vi "Teleop.vi"(10 "Match Info":T2={"Autonomous Elapsed Seconds"=0.0, "TeleOp Elapsed Seconds"=0.0, "Disabled Elapsed Seconds"=0.0, "Visited Autonomous"=FALSE, "Visited TeleOp"=FALSE, "Visited Disabled"=FALSE, "Autonomous Settings"={"Autonomous Style"=enum."Independent", "VI Refnum"=refnum}}, 11 "Call Context":T3) -> ()   [LabVIEW 2015]
doc: "This VI is called for each TeleOp packet received from the DS where the robot is not disabled. It is often used to read from the joysticks and update I/O or to update setpoints for timed control loops. It should complete and return within 20 milliseconds or it may miss DS packets."
uses:
  <vilib>/Rock Robotics/WPI/DriverStation/WPI_DriverStationDerivedRobotMode.ctl
  <vilib>/Rock Robotics/WPI/DriverStation/WPI_DriverStationMatch Info.ctl
  <vilib>/Rock Robotics/WPI/CAN/TalonSRX/WPI_CANTalonSRX_GlobalStatus.ctl
  <vilib>/Rock Robotics/WPI/CAN/TalonSRX/WPI_CANTalonSRX_APIControlMode.ctl
  <vilib>/Rock Robotics/WPI/CAN/TalonSRX/WPI_CANTalonSRX_BrakeOverride.ctl
  <vilib>/Rock Robotics/WPI/Relay/WPI_RelayValue.ctl
  <vilib>/Rock Robotics/Network Tables/NT Write Boolean.vi
  <vilib>/Rock Robotics/WPI/Utilities/WPI_GetSetVariantRefNum.vi
  <vilib>/Rock Robotics/Network Tables/NT Read Boolean.vi
  <vilib>/Rock Robotics/WPI/Solenoid/WPI_SolenoidSetEnum.vi
  <vilib>/Rock Robotics/Network Tables/NT Write Numeric Array.vi
  <vilib>/Rock Robotics/Network Tables/NT Read Number.vi
  <vilib>/Rock Robotics/WPI/RobotDrive/WPI_RobotDriveArcadeDrive_Standard(NoSaturation).vi
panel:
  out "Encoder Position":dbl
  out "Left":T1
  out "Right":T1
  out "Talon SRX Status 2":T1
  out "Talon SRX Status":T1
  out "POSITION":dbl
  out "Theoretical Position":dbl
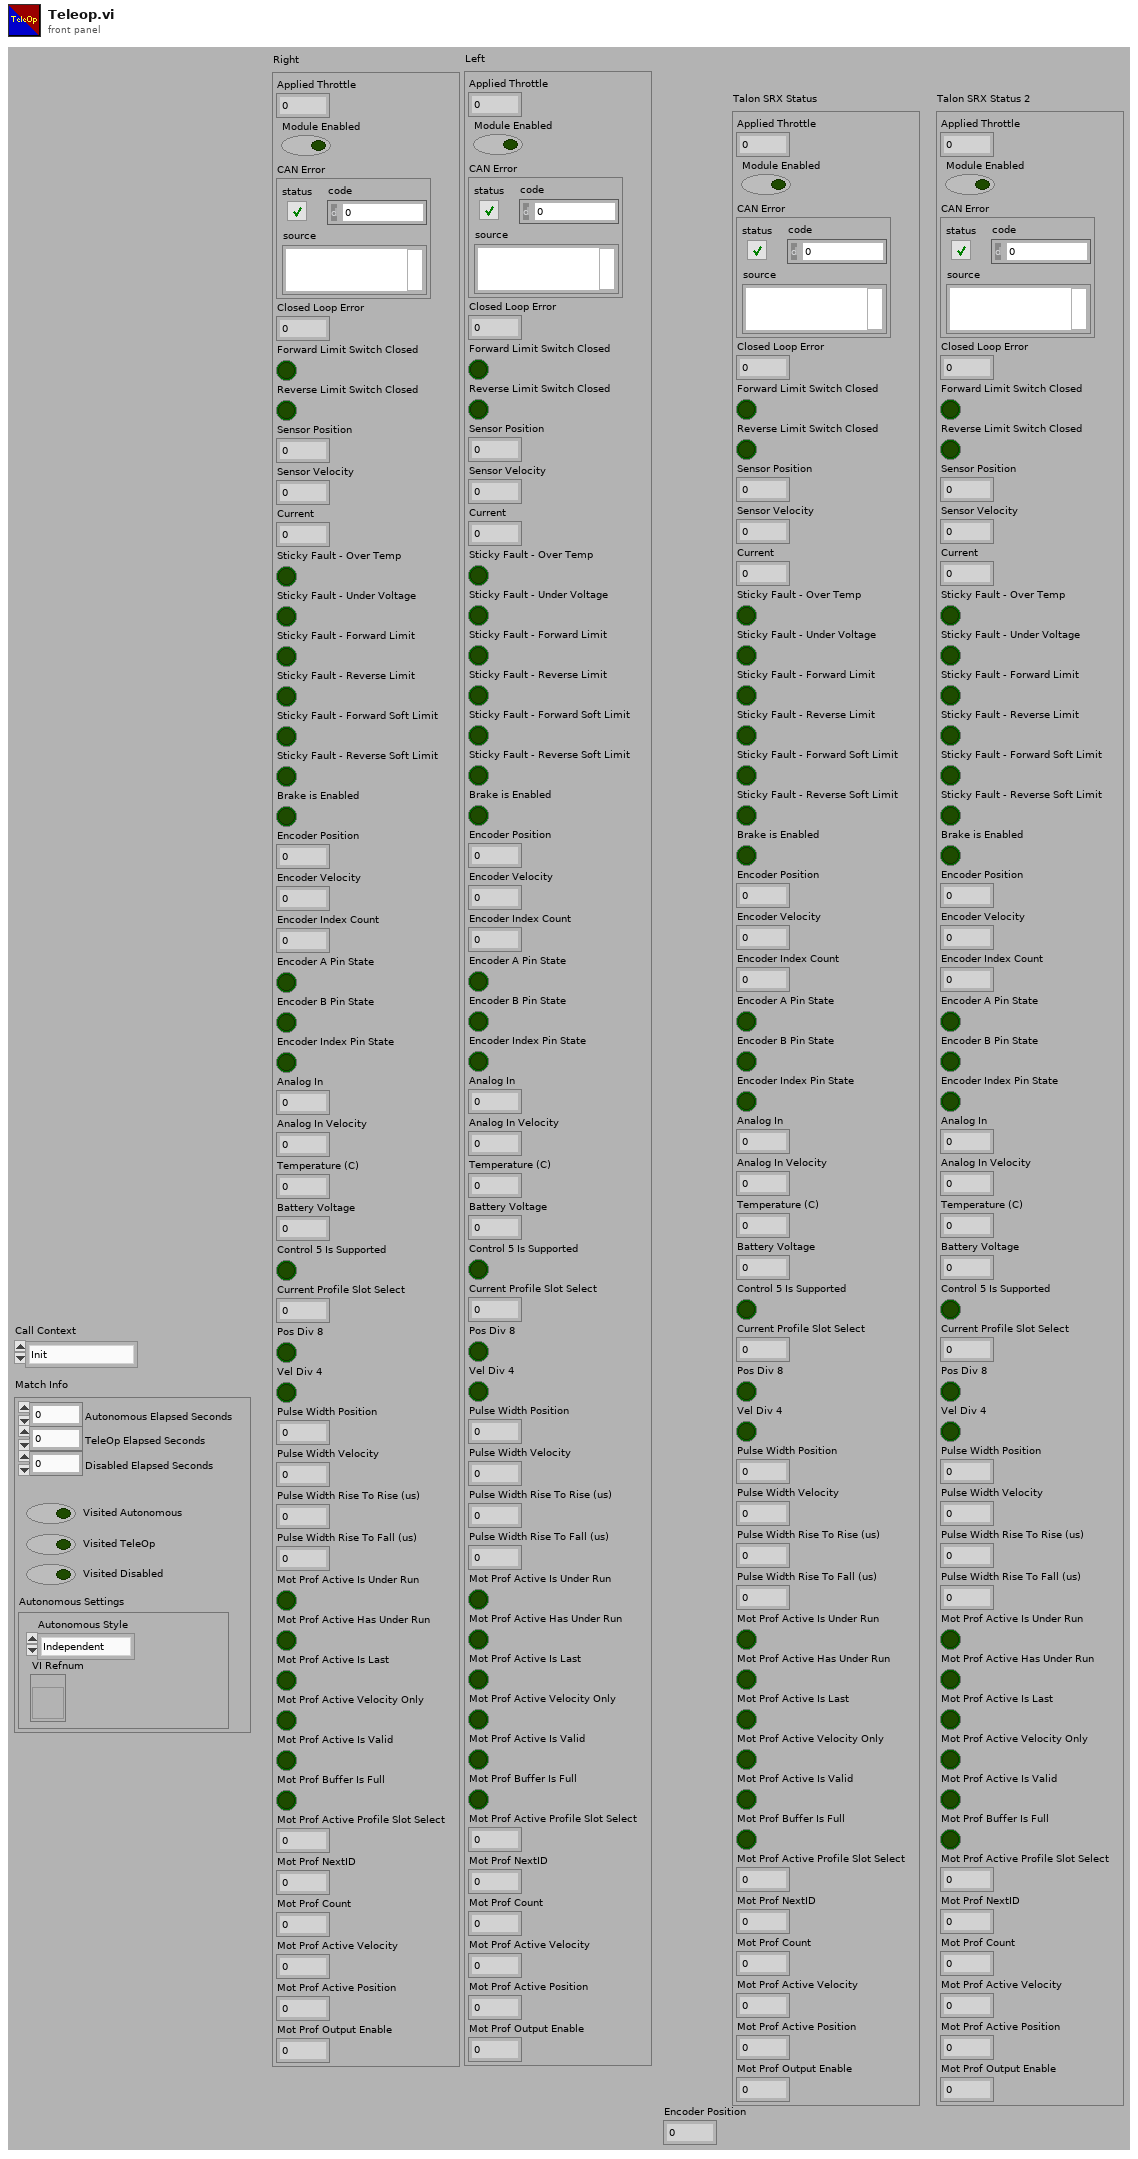
[diagram p1: front panel]
types:
  T1 = typedef "WPI_CANTalonSRX_GlobalStatus.ctl" = cluster{"Applied Throttle":dbl, "Module Enabled":bool, "CAN Error":errorcluster, "Closed Loop Error":dbl, "Forward Limit Switch Closed":bool, "Reverse Limit Switch Closed":bool, "Sensor Position":dbl, "Sensor Velocity":dbl, "Current":dbl, "Sticky Fault - Over Temp":bool, "Sticky Fault - Under Voltage":bool, "Sticky Fault - Forward Limit":bool, "Sticky Fault - Reverse Limit":bool, "Sticky Fault - Forward Soft Limit":bool, "Sticky Fault - Reverse Soft Limit":bool, "Brake is Enabled":bool, "Encoder Position":dbl, "Encoder Velocity":dbl, "Encoder Index Count":dbl, "Encoder A Pin State":bool, "Encoder B Pin State":bool, "Encoder Index Pin State":bool, "Analog In":dbl, "Analog In Velocity":dbl, "Temperature (C)":dbl, "Battery Voltage":dbl, "Control 5 Is Supported":bool, "Current Profile Slot Select":dbl, "Pos Div 8":bool, "Vel Div 4":bool, "Pulse Width Position":i32, "Pulse Width Velocity":i32, "Pulse Width Rise To Rise (us)":i32, "Pulse Width Rise To Fall (us)":i32, "Mot Prof Active Is Under Run":bool, "Mot Prof Active Has Under Run":bool, "Mot Prof Active Is Last":bool, "Mot Prof Active Velocity Only":bool, "Mot Prof Active Is Valid":bool, "Mot Prof Buffer Is Full":bool, "Mot Prof Active Profile Slot Select":i32, "Mot Prof NextID":i32, "Mot Prof Count":i32, "Mot Prof Active Velocity":dbl, "Mot Prof Active Position":dbl, "Mot Prof Output Enable":i32}
  T2 = typedef "WPI_DriverStationMatch Info.ctl" = cluster{"Autonomous Elapsed Seconds":dbl, "TeleOp Elapsed Seconds":dbl, "Disabled Elapsed Seconds":dbl, "Visited Autonomous":bool, "Visited TeleOp":bool, "Visited Disabled":bool, "Autonomous Settings":cluster{"Autonomous Style":enum16{"Iterative", "Independent"}, "VI Refnum":refnum<vi>}}
  T3 = typedef "WPI_DriverStationDerivedRobotMode.ctl" = enum16{"Init", "Execute", "Stop"}
  T4 = typedef "WPI_JoystickDevRef.ctl" = cluster{"Device":T5}
  T5 = typedef "WPI_JoystickDeviceEnum.ctl" = enum16{"USB 0", "USB 1", "USB 2", "USB 3", "USB 4", "USB 5"}
  T6 = cluster{"Axes[0]":dbl, "Axes[1]":dbl, "Axes[2]":dbl, "Axes[3]":dbl, "Axes[4]":dbl, "Axes[5]":dbl, "Axes[6]":dbl, "Axes[7]":dbl, "Axes[8]":dbl}
  T7 = cluster{"Buttons[0]":bool, "Buttons[1]":bool, "Buttons[2]":bool, "Buttons[3]":bool, "Buttons[4]":bool, "Buttons[5]":bool, "Buttons[6]":bool, "Buttons[7]":bool, "Buttons[8]":bool}
  T8 = typedef "WPI_RelayValue.ctl" = enum16{"Off", "On", "Forward", "Reverse"}
  T9 = typedef "WPI_ServoDeviceRef.ctl" = cluster{"DeviceStatus":errorcluster, "PWM Channel":T10, "DeadBand":T11}
  T10 = typedef "FPGA_DIOPWMChannel.ctl" = enum8{"PWM 0", "PWM 1", "PWM 2", "PWM 3", "PWM 4", "PWM 5", "PWM 6", "PWM 7", "PWM 8", "PWM 9", "PWM MXP 0", "PWM MXP 1", "PWM MXP 2", "PWM MXP 3", "PWM MXP 4", "PWM MXP 5", "PWM MXP 6", "PWM MXP 7", "PWM MXP 8", "PWM MXP 9", "Invalid"}
  T11 = typedef "WPI_PWMDeadband.ctl" = cluster{"Name":string, "maxPositivePwm":i32, "minPositivePwm":i32, "centerPwm":i32, "maxNegativePwm":i32, "minNegativePwm":i32, "angularRange":u16}
  T12 = typedef "WPI_SolenoidDevRef.ctl" = cluster{"DevStatus":errorcluster, "Pneumatics Control Module":u8, "Forward Solenoid Channel":T13, "Reverse Solenoid Channel":T13}
  T13 = typedef "WPI_SolenoidChannel.ctl" = enum8{"Solenoid 0", "Solenoid 1", "Solenoid 2", "Solenoid 3", "Solenoid 4", "Solenoid 5", "Solenoid 6", "Solenoid 7", "Invalid"}
  T14 = typedef "WPI_MotorControlDeviceRef.ctl" = cluster{"DeviceStatus":errorcluster, "Type":T15, "PWM":cluster{"PWM Channel":T10, "DeadBand":T11}, "CAN":cluster{"Device Number":u8, "Control Mode":T16, "Semaphore":T17, "Max Vout":dbl, "TalonSRX Control Mode":T18}, "Invert":bool}
  T15 = typedef "WPI_MotorControlType.ctl" = enum16{"PWM", "CAN", "CANTalonSRX"}
  T16 = typedef "WPI_CANJaguar_ControlMode.ctl" = enum8{"Percent VBus", "Current", "Speed", "Position", "Voltage"}
  T17 = typedef "Semaphore RefNum" = refnum<k1>
  T18 = typedef "WPI_CANTalonSRX_APIControlMode.ctl" = enum8{"Percent VBus", "Speed", "Position", "Slave", "Unchanged / Invalid", "Voltage Compensation", "Current", "Motion Profile"}
  T19 = typedef "WPI_CANTalonSRX_BrakeOverride.ctl" = enum8{"No Override", "Override to Coast", "Override to Brake"}
  T20 = typedef "WPI_RobotDriveDevRef.ctl" = cluster{"DevStatus":errorcluster, "Motors[]":T14[], "Square Inputs":bool, "Max Output":dbl}
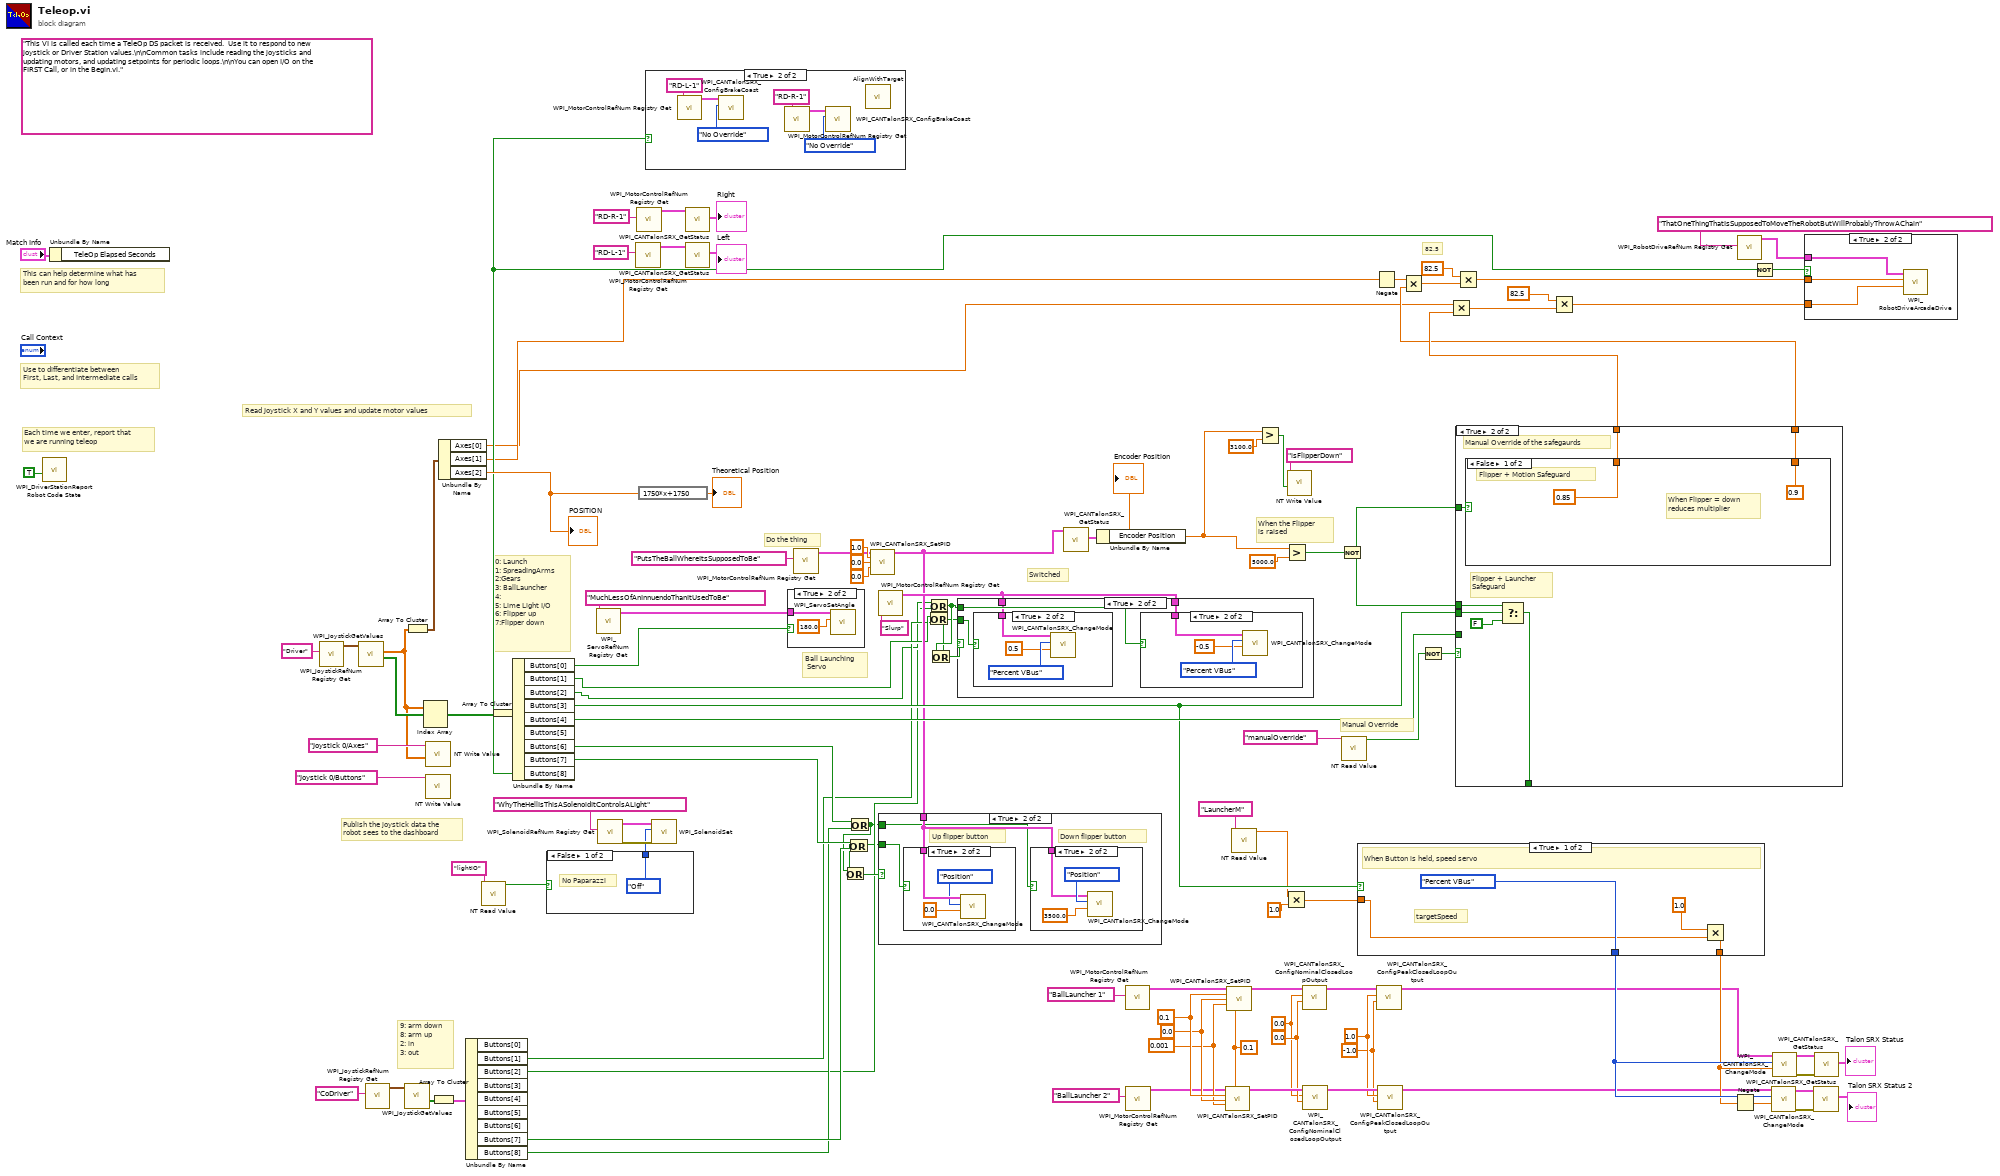
[diagram p0: block diagram]
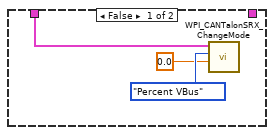
[diagram p7: hidden frame]
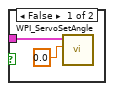
[diagram p10: hidden frame]
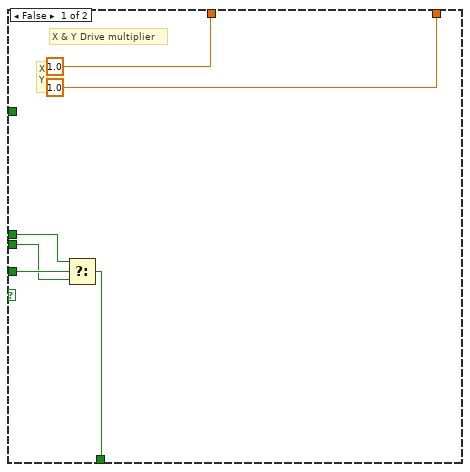
[diagram p11: hidden frame]
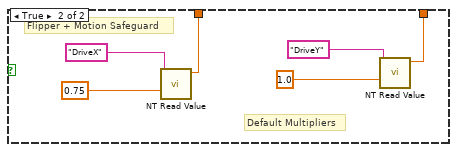
[diagram p12: hidden frame]
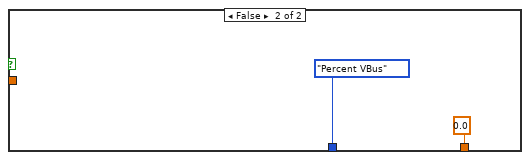
[diagram p13: hidden frame]
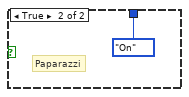
[diagram p14: hidden frame]
diagram:
  w33 = -1.0 ("Reverse Peak Output")
  w34 = 1.0 ("Forward Peak Output")
  w36 = 0.0 ("Reverse Nominal Output")
  w35 = 0.0 ("Forward Nominal Output")
  w32 = 0.1 ("F")
  w45 = 0.001 ("D")
  w46 = 0.0 ("I")
  w47 = 0.1 ("P")
  (unwired) "This VI is called each time a TeleOp DS packet is received.  Use it to respond to new joystick or Driver Station values.\n\nCommon tasks include reading the joysticks and updating motors, and updating setpoints for periodic loops.\n\nYou can open I/O on the FIRST Call, or in the Begin.vi."
  # "82.5"
  # "9: arm down\n8: arm up\n2: in \n3: out"
  # "Switched"
  # "Ball Launching\n Servo"
  # "Manual Override"
  # "When the Flipper \nis raised"
  # "0: Launch\n1: SpreadingArms\n2:Gears\n3: BallLauncher\n4: \n5: Lime Light I/O\n6: Flipper up\n7:Flipper down"
  # "Do the thing"
  # "Publish the joystick data the\nrobot sees to the dashboard"
  # "Read Joystick X and Y values and update motor values"
  # "Each time we enter, report that\nwe are running teleop"
  # "Use to differentiate between\nFirst, Last, and Intermediate calls"
  # "This can help determine what has\nbeen run and for how long"
  n1 = call <vilib>:"WPI_DriverStationReport Robot Code State.vi"("TeleOp"=TRUE ("Autonomous")) -> ()  [unwired: 10 in, 1 out]
  n2 = Unbundle By Name("Match Info") -> ()  [unwired: 1 out]
  n3 = call <vilib>:"WPI_JoystickRefNum Registry Get.vi"("refnum name"="Driver") -> ("JoystickDevRef"=w73:T4)  [unwired: 9 in, 1 out]
  n4 = call <vilib>:"WPI_JoystickGetValues.vi"("JoystickDevRef"=w73) -> ("Buttons"=w70:bool[], "Axes"=w69:dbl[])  [unwired: 6 in, 3 out]
  n5 = call <vilib>:"WPI_JoystickRefNum Registry Get.vi"("refnum name"="CoDriver") -> ("JoystickDevRef"=w21:T4)  [unwired: 9 in, 1 out]
  n6 = call <vilib>:"WPI_JoystickGetValues.vi"("JoystickDevRef"=w21) -> ("Buttons"=w19:bool[])  [unwired: 6 in, 4 out]
  n7 = Array To Cluster(array=w69) -> (cluster=w107:T6)
  n8 = Index Array(array=w69) -> ()  [unwired: 2 in, 2 out]
  n9 = call-poly <vilib>:"NT Write Value.vi"("Numeric Array"=w69, "Name"="Joystick 0/Axes") -> ()  [unwired: 9 in, 1 out]
  n10 = call-poly <vilib>:"NT Write Value.vi"("Name"="Joystick 0/Buttons") -> ()  [unwired: 10 in, 1 out]
  n11 = Array To Cluster(array=w19) -> (cluster=w18:T7)
  n12 = Unbundle By Name(w107) -> ("Axes[0]"=w1:dbl, "Axes[1]"=w2:dbl, "Axes[2]"=w62:dbl)
  "POSITION" <- w62
  n13 = Unbundle By Name(w18) -> ("Buttons[1]"=w12:bool, "Buttons[2]"=w10:bool, "Buttons[7]"=w16:bool, "Buttons[8]"=w14:bool)  [unwired: 5 out]
  n14 = call-poly <vilib>:"NT Read Value.vi"("Name"="lightIO") -> ("Boolean"=w78:bool)  [unwired: 9 in, 1 out]
  n15 = Array To Cluster(array=w70) -> (cluster=w108:T7)
  n16 = Unbundle By Name(w108) -> ("Buttons[0]"=w64:bool, "Buttons[1]"=w13:bool, "Buttons[2]"=w11:bool, "Buttons[3]"=w67:bool, "Buttons[4]"=w68:bool, "Buttons[6]"=w15:bool, "Buttons[7]"=w17:bool, "Buttons[8]"=w4:bool)  [unwired: 1 out]
  n17 = case shown="False" w78 {
    tunnel: [WPI_RelayValue."Off" ("RelayValue") WPI_RelayValue."On" ("RelayValue")] -> w103
    frame False {
      # "No Paparazzi"
    }
    frame True {
      # "Paparazzi"
    }
  }
  n18 = call <vilib>:"WPI_ServoRefNum Registry Get.vi"("refnum name"="MuchLessOfAnInnuendoThanItUsedToBe") -> ("ServoDeviceRef"=w65:T9)  [unwired: 9 in, 1 out]
  n19 = call <vilib>:"WPI_SolenoidRefNum Registry Get.vi"("refnum name"="WhyTheHellIsThisASolenoidItControlsALight") -> ("error out"=w105:errorcluster, "SolenoidDevRef"=w59:T12)  [unwired: 9 in]
  n20 = call <vilib>:"WPI_MotorControlRefNum Registry Get.vi"("refnum name"="RD-L-1") -> ("MotorControlDevRef"=w77:T14)  [unwired: 9 in, 1 out]
  n21 = call <vilib>:"WPI_MotorControlRefNum Registry Get.vi"("refnum name"="RD-R-1") -> ("MotorControlDevRef"=w75:T14)  [unwired: 9 in, 1 out]
  n22 = expression code="1750*x+1750"(w62) -> (→"Theoretical Position":dbl)
  n23 = case shown="True" w4 {
    frame False {
    }
    frame True {
      n24 = call <vilib>:"WPI_MotorControlRefNum Registry Get.vi"("refnum name"="RD-L-1") -> ("MotorControlDevRef"=w119:T14)  [unwired: 9 in, 1 out]
      n25 = call <vilib>:"WPI_CANTalonSRX_ConfigBrakeCoast.vi"("Brake / Coast Mode"=WPI_CANTalonSRX_BrakeOverride."No Override", "CAN Talon SRX Ref"=w119) -> ()  [unwired: 8 in, 2 out]
      n26 = call <vilib>:"WPI_MotorControlRefNum Registry Get.vi"("refnum name"="RD-R-1") -> ("MotorControlDevRef"=w117:T14)  [unwired: 9 in, 1 out]
      n27 = call <vilib>:"WPI_CANTalonSRX_ConfigBrakeCoast.vi"("Brake / Coast Mode"=WPI_CANTalonSRX_BrakeOverride."No Override", "CAN Talon SRX Ref"=w117) -> ()  [unwired: 8 in, 2 out]
      n28 = call "AlignWithTarget.vi"() -> ()  [unwired: 12 in]
    }
  }
  n29 = call-poly <vilib>:"WPI_SolenoidSet.vi"("error in (no error)"=w105, "Value"=w103, "SolenoidDevRef"=w59) -> ()  [unwired: 7 in, 2 out]
  n30 = call <vilib>:"WPI_CANTalonSRX_GetStatus.vi"("CAN Talon SRX Ref"=w75) -> ("Talon SRX Status"=→"Right":T1)  [unwired: 8 in, 2 out]
  n31 = call <vilib>:"WPI_CANTalonSRX_GetStatus.vi"("CAN Talon SRX Ref"=w77) -> ("Talon SRX Status"=→"Left":T1)  [unwired: 8 in, 2 out]
  n32 = case shown="True" w64 {
    tunnel: w65 -> [w121 w124]
    frame False {
      n33 = call <vilib>:"WPI_ServoSetAngle.vi"("Angle"=0.0 ("Position"), "ServoDeviceRef"=w121) -> ()  [unwired: 8 in, 2 out]
    }
    frame True {
      n34 = call <vilib>:"WPI_ServoSetAngle.vi"("Angle"=180.0 ("Position"), "ServoDeviceRef"=w124) -> ()  [unwired: 8 in, 2 out]
    }
  }
  n35 = call <vilib>:"WPI_MotorControlRefNum Registry Get.vi"("refnum name"="PutsTheBallWhereItsSupposedToBe") -> ("MotorControlDevRef"=w50:T14)  [unwired: 9 in, 1 out]
  n36 = Or(x=w17, y=w16) -> (x .or. y?=w6:bool)
  n37 = Or(x=w15, y=w14) -> (x .or. y?=w7:bool)
  n38 = Or(x=w7, y=w6) -> (x .or. y?=w56:bool)
  n39 = call <vilib>:"WPI_CANTalonSRX_SetPID.vi"("CAN Talon SRX Ref"=w50, "P"=1.0, "I"=0.0, "D"=0.0) -> ("CAN Talon SRX Ref"=w49:T14)  [unwired: 10 in, 1 out]
  n40 = call <vilib>:"WPI_MotorControlRefNum Registry Get.vi"("refnum name"="Slurp") -> ("MotorControlDevRef"=w60:T14)  [unwired: 9 in, 1 out]
  n41 = case shown="True" w56 {
    tunnel: w49 -> [_ w127]
    tunnel: w7 -> [_ w126]
    tunnel: w6 -> [_ w125]
    frame False {
    }
    frame True {
      # "Down flipper button"
      # "Up flipper button"
      n42 = case shown="True" w125 {
        tunnel: w127 -> [_ w133]
        frame False {
        }
        frame True {
          n43 = call <vilib>:"WPI_CANTalonSRX_ChangeMode.vi"("Output"=0.0, "Control Mode"=WPI_CANTalonSRX_APIControlMode."Position", "CAN Talon SRX Ref"=w133) -> ()  [unwired: 7 in, 2 out]
        }
      }
      n44 = case shown="True" w126 {
        tunnel: w127 -> [_ w128]
        frame False {
        }
        frame True {
          n45 = call <vilib>:"WPI_CANTalonSRX_ChangeMode.vi"("Output"=3500.0, "Control Mode"=WPI_CANTalonSRX_APIControlMode."Position", "CAN Talon SRX Ref"=w128) -> ()  [unwired: 7 in, 2 out]
        }
      }
    }
  }
  n46 = Or(x=w13, y=w12) -> (x .or. y?=w3:bool)
  n47 = Or(x=w11, y=w10) -> (x .or. y?=w5:bool)
  n48 = Or(x=w5, y=w3) -> (x .or. y?=w61:bool)
  n49 = case shown="True" w61 {
    tunnel: w5 -> [_ w140]
    tunnel: w3 -> [_ w139]
    tunnel: w60 -> [w134 w138]
    tunnel: w60 -> [_ w137]
    frame False {
      n50 = call <vilib>:"WPI_CANTalonSRX_ChangeMode.vi"("Output"=0.0, "Control Mode"=WPI_CANTalonSRX_APIControlMode."Percent VBus", "CAN Talon SRX Ref"=w134) -> ()  [unwired: 7 in, 2 out]
    }
    frame True {
      n51 = case shown="True" w139 {
        tunnel: w138 -> [_ w146]
        frame False {
        }
        frame True {
          n52 = call <vilib>:"WPI_CANTalonSRX_ChangeMode.vi"("Output"=0.5, "Control Mode"=WPI_CANTalonSRX_APIControlMode."Percent VBus", "CAN Talon SRX Ref"=w146) -> ()  [unwired: 7 in, 2 out]
        }
      }
      n53 = case shown="True" w140 {
        tunnel: w137 -> [_ w141]
        frame False {
        }
        frame True {
          n54 = call <vilib>:"WPI_CANTalonSRX_ChangeMode.vi"("Output"=-0.5, "Control Mode"=WPI_CANTalonSRX_APIControlMode."Percent VBus", "CAN Talon SRX Ref"=w141) -> ()  [unwired: 7 in, 2 out]
        }
      }
    }
  }
  n55 = call <vilib>:"WPI_CANTalonSRX_GetStatus.vi"("CAN Talon SRX Ref"=w49) -> ("Talon SRX Status"=w101:T1)  [unwired: 8 in, 2 out]
  n56 = Unbundle By Name(w101) -> ("Encoder Position"=w48:dbl)
  "Encoder Position" <- w48
  n57 = call <vilib>:"WPI_MotorControlRefNum Registry Get.vi"("refnum name"="BallLauncher 1") -> ("MotorControlDevRef"=w44:T14)  [unwired: 9 in, 1 out]
  n58 = call <vilib>:"WPI_MotorControlRefNum Registry Get.vi"("refnum name"="BallLauncher 2") -> ("MotorControlDevRef"=w43:T14)  [unwired: 9 in, 1 out]
  n59 = call <vilib>:"WPI_CANTalonSRX_SetPID.vi"("CAN Talon SRX Ref"=w43, "P"=w47, "I"=w46, "D"=w45, "F"=w32) -> ("CAN Talon SRX Ref"=w38:T14)  [unwired: 9 in, 1 out]
  n60 = call <vilib>:"WPI_CANTalonSRX_SetPID.vi"("CAN Talon SRX Ref"=w44, "P"=w47, "I"=w46, "D"=w45, "F"=w32) -> ("CAN Talon SRX Ref"=w39:T14)  [unwired: 9 in, 1 out]
  n61 = call-poly <vilib>:"NT Read Value.vi"("Name"="LauncherM") -> ("Numeric"=w9:dbl)  [unwired: 9 in, 1 out]
  n62 = Greater?(x=w48, y=3100.0) -> (0:w82:bool)
  n63 = Multiply(x=w9, y=1.0) -> (x*y=w80:dbl)
  n64 = Greater?(x=w48, y=5000.0) -> (0:w91:bool)
  n65 = call-poly <vilib>:"NT Write Value.vi"("Boolean"=w82, "Name"="isFlipperDown") -> ()  [unwired: 9 in, 1 out]
  n66 = call <vilib>:"WPI_CANTalonSRX_ConfigNominalClosedLoopOutput.vi"("Reverse Nominal Output"=w36, "Forward Nominal Output"=w35, "CAN Talon SRX Ref"=w39) -> ("CAN Talon SRX Ref"=w40:T14)  [unwired: 7 in, 1 out]
  n67 = call <vilib>:"WPI_CANTalonSRX_ConfigNominalClosedLoopOutput.vi"("Reverse Nominal Output"=w36, "Forward Nominal Output"=w35, "CAN Talon SRX Ref"=w38) -> ("CAN Talon SRX Ref"=w37:T14)  [unwired: 7 in, 1 out]
  n68 = Not(x=w91) -> (.not. x?=w90:bool)
  n69 = call-poly <vilib>:"NT Read Value.vi"("Name"="manualOverride") -> ("Boolean"=w84:bool)  [unwired: 9 in, 1 out]
  n70 = case shown="True" w67 {
    tunnel: [w149 0.0] -> w41
    tunnel: [WPI_CANTalonSRX_APIControlMode."Percent VBus" ("Control Mode") WPI_CANTalonSRX_APIControlMode."Percent VBus" ("Control Mode")] -> w87
    tunnel: w80 -> [w147 _]
    frame True {
      # "targetSpeed"
      # "When Button is held, speed servo"
      n71 = Multiply(x=1.0, y=w147) -> (x*y=w149:dbl)
    }
    frame False {
    }
  }
  n72 = Negate(x=w2) -> (-x=w58:dbl)
  n73 = call <vilib>:"WPI_CANTalonSRX_ConfigPeakClosedLoopOutput.vi"("Reverse Peak Output"=w33, "Forward Peak Output"=w34, "CAN Talon SRX Ref"=w40) -> ("CAN Talon SRX Ref"=w31:T14)  [unwired: 7 in, 1 out]
  n74 = call <vilib>:"WPI_CANTalonSRX_ConfigPeakClosedLoopOutput.vi"("Reverse Peak Output"=w33, "Forward Peak Output"=w34, "CAN Talon SRX Ref"=w37) -> ("CAN Talon SRX Ref"=w30:T14)  [unwired: 7 in, 1 out]
  n75 = Not(x=w84) -> (.not. x?=w71:bool)
  n76 = case shown="True" w71 {
    tunnel: [1.0 ("Numeric") w165] -> w89
    tunnel: [1.0 ("Numeric") w164] -> w88
    tunnel: w90 -> [w153 w162]
    tunnel: w67 -> [w155 w161]
    tunnel: [w154 w160] -> _
    tunnel: w90 -> [_ w159]
    tunnel: w68 -> [w156 _]
    frame False {
      # "X\nY"
      # "X & Y Drive multiplier"
      n77 = Select(t=w153, s=w156, f=w155) -> (s? t:f=w154:bool)
    }
    frame True {
      # "Flipper + Launcher\nSafeguard"
      # "Manual Override of the safegaurds"
      n78 = case shown="False" w159 {
        tunnel: [0.85 ("Numeric") w171] -> w165
        tunnel: [0.9 ("Numeric") w168] -> w164
        frame False {
          # "When Flipper = down\nreduces multiplier"
          # "Flipper + Motion Safeguard"
        }
        frame True {
          # "Default Multipliers"
          # "Flipper + Motion Safeguard"
          n79 = call-poly <vilib>:"NT Read Value.vi"("Default Value"=0.75, "Name"="DriveX") -> ("Numeric"=w171:dbl)  [unwired: 8 in, 1 out]
          n80 = call-poly <vilib>:"NT Read Value.vi"("Default Value"=1.0, "Name"="DriveY") -> ("Numeric"=w168:dbl)  [unwired: 8 in, 1 out]
        }
      }
      n81 = Select(t=w162, s=w161, f=FALSE) -> (s? t:f=w160:bool)
    }
  }
  n82 = Multiply(x=w58, y=w88) -> (x*y=w29:dbl)
  n83 = Multiply(x=w1, y=w89) -> (x*y=w25:dbl)
  n84 = Multiply(x=82.5, y=w29) -> (x*y=w27:dbl)
  n85 = Multiply(x=82.5, y=w25) -> (x*y=w24:dbl)
  n86 = Negate(x=w41) -> (-x=w42:dbl)
  n87 = call <vilib>:"WPI_RobotDriveRefNum Registry Get.vi"("refnum name"="ThatOneThingThatIsSupposedToMoveTheRobotButWillProbablyThrowAChain") -> ("RobotDriveDevRef"=w52:T20)  [unwired: 9 in, 1 out]
  n88 = Not(x=w4) -> (.not. x?=w51:bool)
  n89 = call <vilib>:"WPI_CANTalonSRX_ChangeMode.vi"("Output"=w42, "Control Mode"=w87, "CAN Talon SRX Ref"=w30) -> ("error out"=w96:errorcluster, "CAN Talon SRX Ref"=w95:T14)  [unwired: 7 in]
  n90 = call <vilib>:"WPI_CANTalonSRX_ChangeMode.vi"("Output"=w41, "Control Mode"=w87, "CAN Talon SRX Ref"=w31) -> ("error out"=w86:errorcluster, "CAN Talon SRX Ref"=w97:T14)  [unwired: 7 in]
  n91 = case shown="True" w51 {
    tunnel: w52 -> [_ w176]
    tunnel: w24 -> [_ w175]
    tunnel: w27 -> [_ w174]
    frame False {
    }
    frame True {
      n92 = call-poly <vilib>:"WPI_RobotDriveArcadeDrive.vi"("Y axis value"=w175, "X axis value"=w174, "RobotDriveDevRef"=w176) -> ()  [unwired: 6 in, 3 out]
    }
  }
  n93 = call <vilib>:"WPI_CANTalonSRX_GetStatus.vi"("error in (no error)"=w96, "CAN Talon SRX Ref"=w95) -> ("Talon SRX Status"=→"Talon SRX Status 2":T1)  [unwired: 7 in, 2 out]
  n94 = call <vilib>:"WPI_CANTalonSRX_GetStatus.vi"("error in (no error)"=w86, "CAN Talon SRX Ref"=w97) -> ("Talon SRX Status"=→"Talon SRX Status":T1)  [unwired: 7 in, 2 out]
